vi "fit_data.vi"(8 "error in (no error)":errorcluster, 11 "Plots in":refnum<class "Plots.lvclass">) -> (0 "error out":errorcluster, 3 "Plots out":refnum<class "Plots.lvclass">)   [LabVIEW 2018, in "Plots.lvclass"]
doc: "fits the data"
uses:
  Plots.lvclass
  <vilib>/Analysis/6fits.llb/Curve Fitting Criteria.ctl
  <vilib>/Analysis/6fits.llb/Confidence Interval (Linear).vi
  <vilib>/Analysis/6fits.llb/Confidence Interval (Polynomial).vi
  <vilib>/Analysis/NI_AALPro.lvlib
panel:
  out "delta intercept":dbl
  out "Lower Bound":dbl[](array[numeric])
  out "Upper Bound":dbl[](array[numeric])
  out "RMSE":dbl
  out "residue":dbl
  out "intercept":dbl
  out "slope":dbl
  out "Best Linear Fit":dbl[](array[numeric])
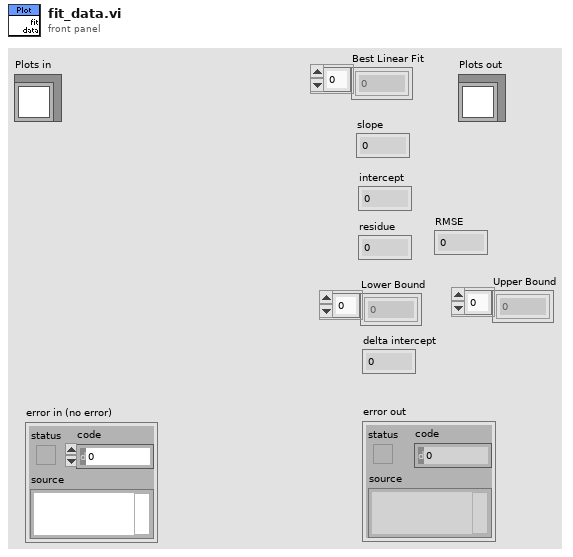
[diagram p1: front panel]
types:
  T1 = typedef "NI_AALPro.lvlib/Curve Fitting Criteria.ctl" = u16
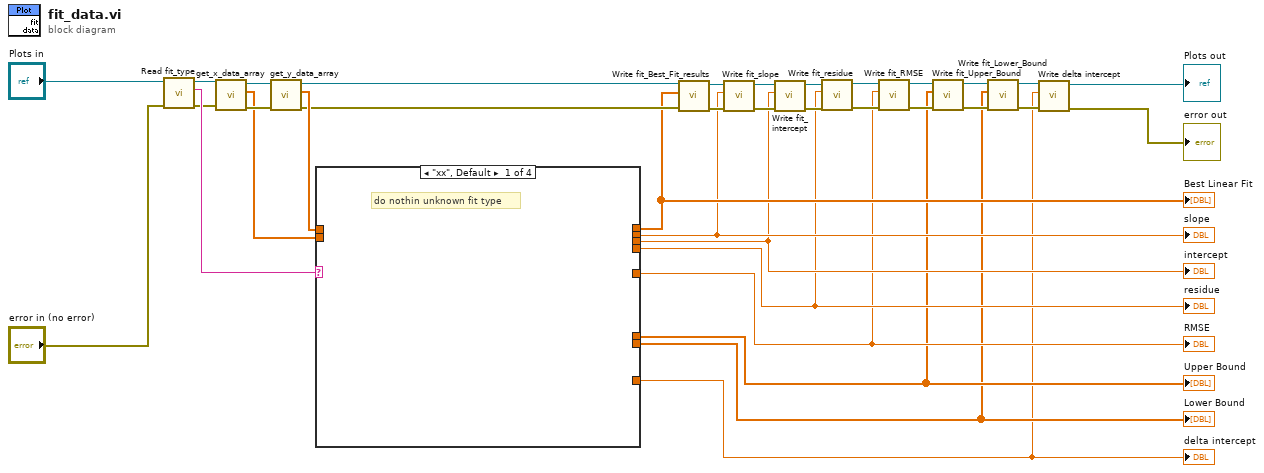
[diagram p0: block diagram]
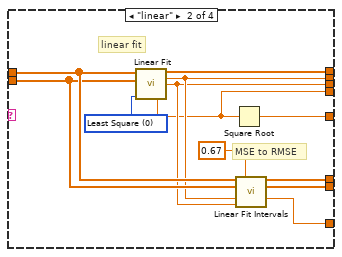
[diagram p2: hidden frame]
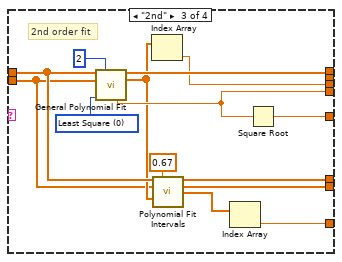
[diagram p3: hidden frame]
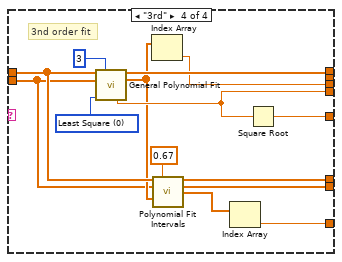
[diagram p4: hidden frame]
diagram:
  n1 = call-dynamic "Read fit_type.vi"("error in (no error)"="error in (no error)", "Plots in"="Plots in") -> ("error out"=w31:errorcluster, "fit_type"=w33:string, "Plots out"=w32:refnum<class "Plots.lvclass">)  [unwired: 7 in]
  n2 = call-dynamic "get_x_data_array.vi"("error in (no error)"=w31, "Plots in"=w32) -> ("error out"=w29:errorcluster, "x-Array"=w28:dbl[], "Plots out"=w30:refnum<class "Plots.lvclass">)  [unwired: 7 in]
  n3 = call-dynamic "get_y_data_array.vi"("error in (no error)"=w29, "Plots in"=w30) -> ("error out"=w25:errorcluster, "y-Array"=w27:dbl[], "Plots out"=w26:refnum<class "Plots.lvclass">)  [unwired: 7 in]
  n4 = case shown="\"xx\", Default" w33 {
    tunnel: w28 -> [_ w44 w48 w62]
    tunnel: w27 -> [_ w45 w56 w70]
    tunnel: [_ w46 w59 w73] -> w18
    tunnel: [_ w43 _ _] -> w17
    tunnel: [_ w42 w51 w65] -> w16
    tunnel: [_ w38 w58 w72] -> w15
    tunnel: [_ w41 w49 w63] -> w1
    tunnel: [_ w40 w55 w69] -> w5
    tunnel: [_ w39 w54 w68] -> w4
    tunnel: [_ w37 w57 w71] -> w6
    frame "xx", Default {
      # "do nothin unknown fit type"
    }
    frame "linear" {
      w47 = T1 0 items=["Least Square", "Least Absolute Residual", "Bisquare"] ("method")
      # "MSE to RMSE"
      # "linear fit"
      n5 = call <vilib>:"Linear Fit.vi"("Y"=w45, "X"=w44, "method"=w47) -> ("Best Linear Fit"=w46:dbl[], "slope"=w43:dbl, "intercept"=w42:dbl, "residue"=w38:dbl)  [unwired: 8 in, 1 out]
      n6 = Square Root(x=w38) -> (sqrt(x)=w37:dbl)
      n7 = call-poly <vilib>:"Linear Fit Intervals.vi"("Y"=w45, "confidence level"=0.67, "X"=w44, "slope"=w43, "intercept"=w42) -> ("Upper Bound"=w40:dbl[], "Lower Bound"=w39:dbl[], "delta intercept"=w41:dbl)  [unwired: 6 in, 2 out]
    }
    frame "2nd" {
      w61 = T1 0 items=["Least Square", "Least Absolute Residual", "Bisquare"] ("method")
      # "2nd order fit"
      n8 = call <vilib>:"General Polynomial Fit.vi"("Y"=w56, "polynomial order"=2, "X"=w48, "method"=w61) -> ("Best Polynomial Fit"=w59:dbl[], "Polynomial Coefficients"=w52:dbl[], "residue"=w58:dbl)  [unwired: 8 in, 1 out]
      n9 = Index Array(array=w52) -> (element=w51:dbl)  [unwired: 1 in]
      n10 = call-poly <vilib>:"Polynomial Fit Intervals.vi"("Y"=w56, "confidence level"=0.67, "X"=w48, "Polynomial Coefficients"=w52) -> ("Upper Bound"=w55:dbl[], "Lower Bound"=w54:dbl[], "Delta Polynomial Coefficients"=w50:dbl[])  [unwired: 8 in, 1 out]
      n11 = Index Array(array=w50) -> (element=w49:dbl)  [unwired: 1 in]
      n12 = Square Root(x=w58) -> (sqrt(x)=w57:dbl)
    }
    frame "3rd" {
      w75 = T1 0 items=["Least Square", "Least Absolute Residual", "Bisquare"] ("method")
      # "3nd order fit"
      n13 = call <vilib>:"General Polynomial Fit.vi"("Y"=w70, "polynomial order"=3, "X"=w62, "method"=w75) -> ("Best Polynomial Fit"=w73:dbl[], "Polynomial Coefficients"=w66:dbl[], "residue"=w72:dbl)  [unwired: 8 in, 1 out]
      n14 = Index Array(array=w66) -> (element=w65:dbl)  [unwired: 1 in]
      n15 = call-poly <vilib>:"Polynomial Fit Intervals.vi"("Y"=w70, "confidence level"=0.67, "X"=w62, "Polynomial Coefficients"=w66) -> ("Upper Bound"=w69:dbl[], "Lower Bound"=w68:dbl[], "Delta Polynomial Coefficients"=w64:dbl[])  [unwired: 8 in, 1 out]
      n16 = Index Array(array=w64) -> (element=w63:dbl)  [unwired: 1 in]
      n17 = Square Root(x=w72) -> (sqrt(x)=w71:dbl)
    }
  }
  "Best Linear Fit" <- w18
  "slope" <- w17
  "intercept" <- w16
  "residue" <- w15
  "RMSE" <- w6
  "Upper Bound" <- w5
  "Lower Bound" <- w4
  "delta intercept" <- w1
  n18 = call-dynamic "Write fit_Best_Fit_results.vi"("error in (no error)"=w25, "fit_Best_Fit_results"=w18, "Plots in"=w26) -> ("error out"=w23:errorcluster, "Plots out"=w24:refnum<class "Plots.lvclass">)  [unwired: 7 in]
  n19 = call-dynamic "Write fit_slope.vi"("error in (no error)"=w23, "fit_slope"=w17, "Plots in"=w24) -> ("error out"=w21:errorcluster, "Plots out"=w22:refnum<class "Plots.lvclass">)  [unwired: 7 in]
  n20 = call-dynamic "Write fit_intercept.vi"("error in (no error)"=w21, "fit_intercept"=w16, "Plots in"=w22) -> ("error out"=w19:errorcluster, "Plots out"=w20:refnum<class "Plots.lvclass">)  [unwired: 7 in]
  n21 = call-dynamic "Write fit_residue.vi"("error in (no error)"=w19, "fit_residue"=w15, "Plots in"=w20) -> ("error out"=w13:errorcluster, "Plots out"=w14:refnum<class "Plots.lvclass">)  [unwired: 7 in]
  n22 = call-dynamic "Write fit_RMSE.vi"("error in (no error)"=w13, "fit_RMSE"=w6, "Plots in"=w14) -> ("error out"=w11:errorcluster, "Plots out"=w12:refnum<class "Plots.lvclass">)  [unwired: 7 in]
  n23 = call-dynamic "Write fit_Upper_Bound.vi"("error in (no error)"=w11, "fit_Upper_Bound"=w5, "Plots in"=w12) -> ("error out"=w9:errorcluster, "Plots out"=w10:refnum<class "Plots.lvclass">)  [unwired: 7 in]
  n24 = call-dynamic "Write fit_Lower_Bound.vi"("error in (no error)"=w9, "fit_Lower_Bound"=w4, "Plots in"=w10) -> ("error out"=w7:errorcluster, "Plots out"=w8:refnum<class "Plots.lvclass">)  [unwired: 7 in]
  n25 = call-dynamic "Write delta intercept.vi"("error in (no error)"=w7, "delta intercept"=w1, "Plots in"=w8) -> ("error out"=→"error out":errorcluster, "Plots out"=→"Plots out":refnum<class "Plots.lvclass">)  [unwired: 7 in]
